vi "Main RT.vi"() -> ()   [LabVIEW 2021]
panel:
  in  "Slide 2":dbl(slide) scale=0.0..10.0
  in  "Slide":dbl(slide) scale=0.0..10.0
  in  "stop":bool
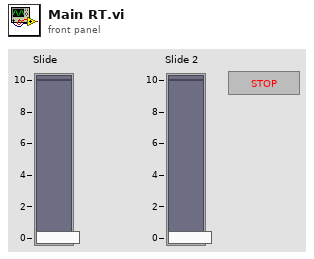
[diagram p1: front panel]
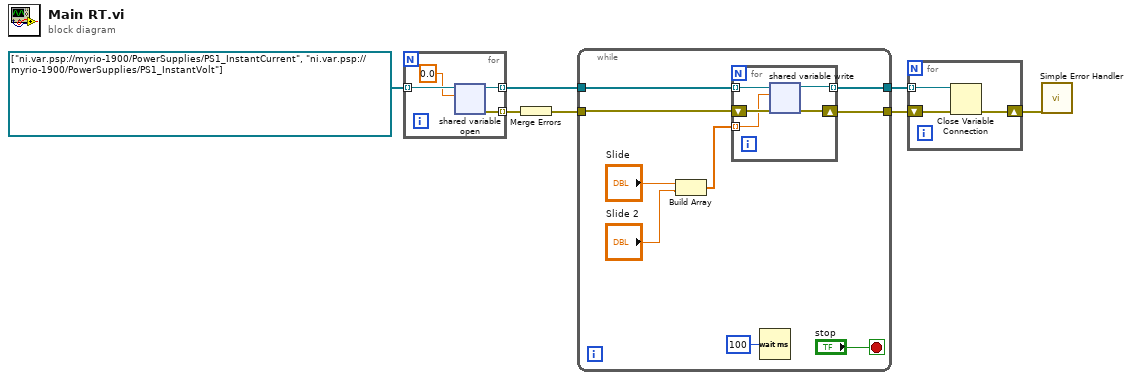
[diagram p0: block diagram]
diagram:
  n1 = for {
    tunnel: [w11] -> w3 mode=indexing
    tunnel: refnum<k21>[] ["ni.var.psp://myrio-1900/PowerSupplies/PS1_InstantCurrent", "ni.var.psp://myrio-1900/PowerSupplies/PS1_InstantVolt"] ("shared variable refnum in") -> [w10] mode=indexing
    tunnel: [w8] -> w5 mode=indexing
    n2 = shared-variable-open(w10, 0.0) -> (w11:refnum<k21>, w8:errorcluster)  [unwired: 2 in]
  }
  n3 = Merge Errors(w5) -> (w6:errorcluster)
  n4 = while {
    tunnel: w3 -> [w18]
    tunnel: w6 -> [w15]
    tunnel: [w17] -> w2
    tunnel: [w16] -> w1
    stop <- "stop" stop-if-true
    n5 = Build Array("Slide", "Slide 2") -> (w13:dbl[])
    n6 = for {
      tunnel: w18 -> [w24] mode=indexing
      tunnel: [w23] -> w17 mode=indexing
      shift-right: [w22] -> w16
      shift-left: w15 -> [w25]
      tunnel: w13 -> [w21] mode=indexing
      n7 = shared-variable-write(w24, w25, w21) -> (w23:refnum<k21>, w22:errorcluster)
    }
    n8 = Wait (ms)(milliseconds to wait=u32 100) -> ()  [unwired: 1 out]
  }
  n9 = for {
    shift-right: [w27] -> w7
    shift-left: w1 -> [w28]
    tunnel: w2 -> [w26] mode=indexing
    n10 = Close Variable Connection(8:w28, 11:w26) -> (0:w27:errorcluster)
  }
  n11 = call <vilib>:"Simple Error Handler.vi"("error in (no error)"=w7) -> ()  [unwired: 4 in, 5 out]
